vi "權限密碼.vi"() -> ()   [LabVIEW 2015]
uses:
  3.SubVI/Read_ini_ArrayStr.vi
panel:
  in  "User":u16(ring) items=["操作員", "工程師", "廠商"]
  in  "New Password":string
  in  "Old Password":string
  in  "Confirm":bool
  in  "Exit":bool
  # "權限密碼"
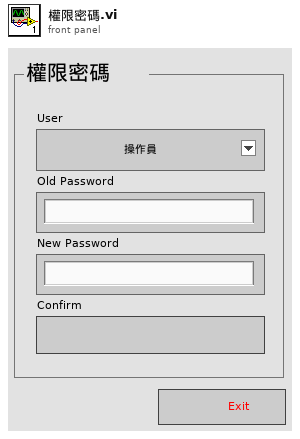
[diagram p1: front panel]
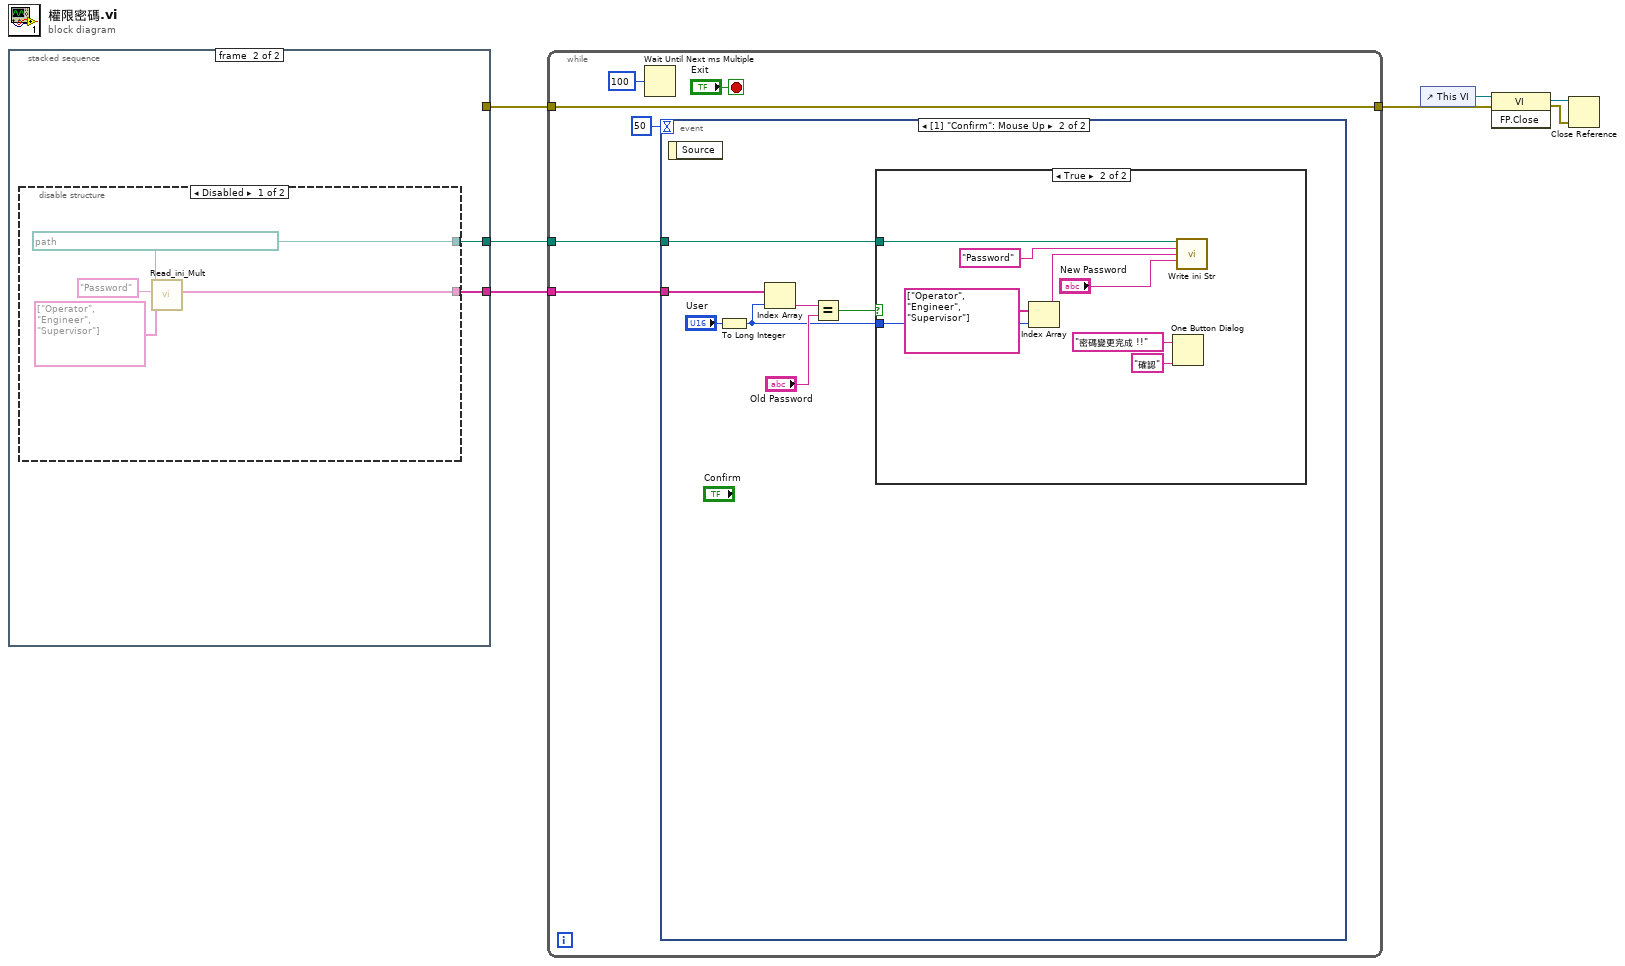
[diagram p0: block diagram]
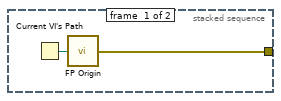
[diagram p2: hidden frame]
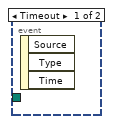
[diagram p4: hidden frame]
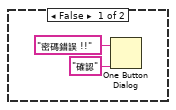
[diagram p5: hidden frame]
diagram:
  n1 = stacked-sequence {
    tunnel: [w8 _] -> w3
    tunnel: [_ w11] -> w2
    tunnel: [_ w10] -> w1
    frame #0 {
      n2 = Current VI's Path() -> (path=w9:path)
      n3 = call "FP Origin.vi"("vi path"=w9) -> ("error out"=w8:errorcluster)
    }
    frame #1 {
      n4 = disable-structure shown="Disabled" {
        disable-tunnel: [w13 _] -> w11
        disable-tunnel: [w12 _] -> w10
        frame Disabled {
          w12 = path "D:/Folding自動機 Data/Recipe/Default.ini" ("configuration file path")
          n5 = call-poly "Read_ini_Mult.vi"("key names"=string[] ["Operator", "Engineer", "Supervisor"], "section"="Password", "configuration file path"=w12) -> ("ArrayValue"=w13:string[])  [unwired: 7 in, 1 out]
        }
        frame Enabled {
        }
      }
    }
  }
  n6 = while {
    tunnel: w3 -> [w18]
    tunnel: [w18] -> w7
    tunnel: w2 -> [w17]
    tunnel: w1 -> [w16]
    stop <- "Exit" stop-if-true
    n7 = Wait Until Next ms Multiple(millisecond multiple=u32 100) -> ()  [unwired: 1 out]
    n8 = event shown="[1] \"Confirm\": Mouse Up" {
      selector: _ -> [_ _]
      dyn-events: _ -> [_ _]
      timeout: 50 -> [_ _]
      tunnel: w17 -> [_ w28]
      tunnel: w16 -> [_ w23]
      event Timeout {
        n9 = event-data() -> ()  [unwired: 1 in, 3 out]
      }
      event "Confirm": Mouse Up {
        n10 = event-data() -> ()  [unwired: 1 in, 1 out]
        n11 = To Long Integer(number="User") -> (32bit integer=w22:i32)
        n12 = Index Array(array=w28, index=w22) -> (element=w26:string)
        n13 = Equal?(x=w26, y="Old Password") -> (x = y?=w24:bool)
        n14 = case shown="True" w24 {
          tunnel: w23 -> [_ w38]
          tunnel: w22 -> [_ w35]
          frame False {
            n15 = One Button Dialog(message="密碼錯誤 !!", button name ("OK")="確認") -> ()  [unwired: 1 out]
          }
          frame True {
            n16 = Index Array(array=string[] ["Operator", "Engineer", "Supervisor"], index=w35) -> (element=w34:string)
            n17 = One Button Dialog(message="密碼變更完成 !!", button name ("OK")="確認") -> ()  [unwired: 1 out]
            n18 = call "Write ini Str.vi"("configuration file path"=w38, "section"="Password", "key"=w34, "value"="New Password") -> ()  [unwired: 11 in, 1 out]
          }
        }
      }
    }
  }
  n19 = control-ref of="This VI"() -> (w6:refnum<vi>)
  n20 = invoke class="VI" method="FP.Close"(reference=w6, error in=w7) -> (reference out=w5:refnum<vi>, error out=w4:errorcluster)  [unwired: 1 in, 1 out]
  n21 = Close Reference(reference=w5, error in (no error)=w4) -> ()  [unwired: 1 out]
